vi "Image Aqq.vi"(3 "Error In":errorcluster, 4 "Img In":T1, 5 "Session In":T2 caption="Camera") -> (0 "Error Out":errorcluster, 1 "Image":T1(plugin-control), 2 "Cam Out":T2)   [LabVIEW 2015]
uses:
  <vilib>/userdefined/High Color/IMAQdx.ctl
  <vilib>/vision/Image Controls.llb/IMAQ Image.ctl
  <vilib>/vision/driver/NI_Vision_Acquisition_Software.lvlib
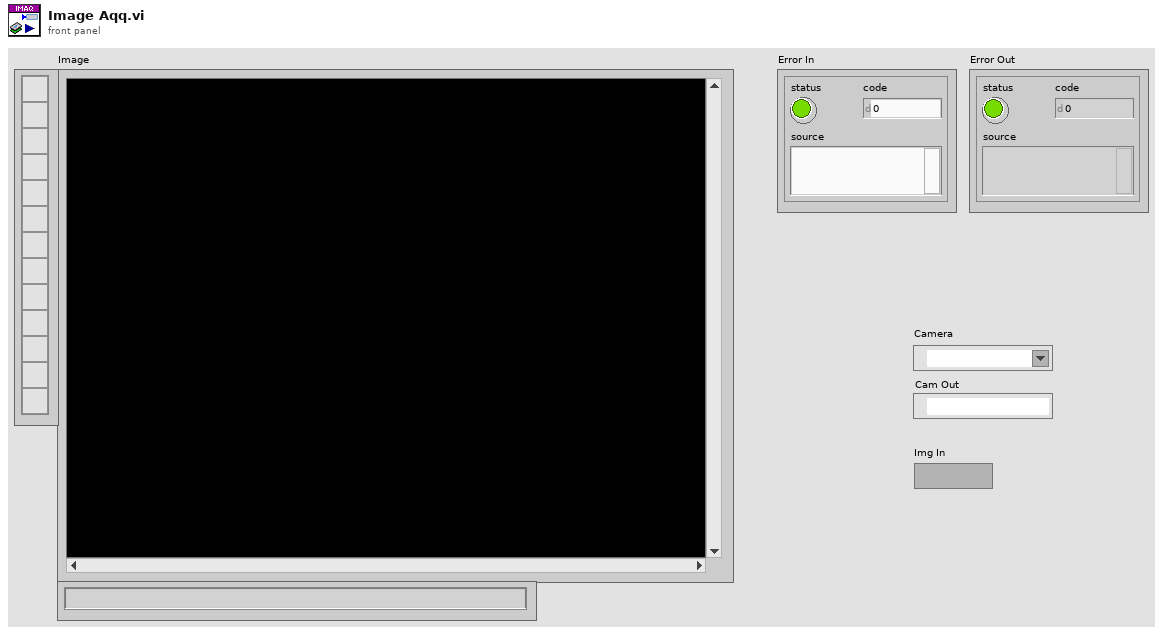
[diagram p1: front panel]
types:
  T1 = typedef "IMAQ Image.ctl" = refnum<image>
  T2 = typedef "IMAQdx.ctl" = refnum<k21>
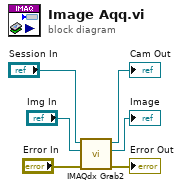
[diagram p0: block diagram]
diagram:
  n1 = call <vilib>:"IMAQdx Grab2.vi"("error in"="Error In", "Image In"="Img In", "Session In"="Session In") -> ("error out"=→"Error Out":errorcluster, "Image Out"=→"Image":T1, "Session Out"=→"Cam Out":T2)  [unwired: 5 in, 1 out]
